vi "Live window-Graph intensity matching.vi"(8 "error in (no error)":errorcluster, 11 "Left/Right":T1) -> (0 "error out":errorcluster)   [LabVIEW 2017]
uses:
  Typedefs/Left-Right enum.ctl
  Globals/gl_Windows Ctrl refs.vi
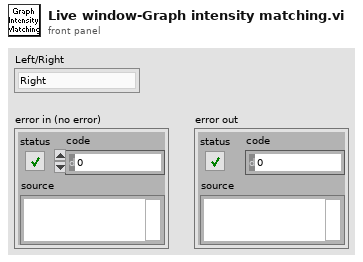
[diagram p1: front panel]
types:
  T1 = typedef "Left-Right enum.ctl" = enum16{"Right", "Left"}
  T2 = typedef "Live window-ctrl refs.ctl" = cluster{"This VI":refnum<vi>, "Pane":refnum<vi>, "Show REF Image Left":refnum<vi>, "Show REF Image Right":refnum<vi>, "Snapshot":refnum<vi>, "Left Image Palette":refnum<vi>, "Right Image Palette":refnum<vi>, "Left Channel":refnum<vi>, "Right Channel":refnum<vi>, "Left image intensity":refnum<vi>, "Right image intensity":refnum<vi>, "Left Image Display":T3, "Right Image Display":T3, "Refresh rate ind (Hz)":refnum<vi>, "Acq rate ind (Hz)":refnum<vi>, "Stop (ind)":refnum<vi>}
  T3 = typedef "Image display ref.ctl" = refnum<vi>
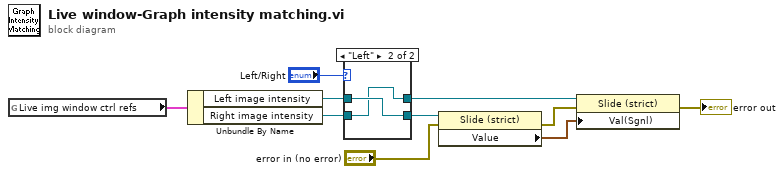
[diagram p0: block diagram]
diagram:
  n1 = global read "gl_Windows Ctrl refs.vi" "Live img window ctrl refs"() -> (w10:T2)
  n2 = Unbundle By Name(w10) -> ("Left image intensity"=w8:refnum<vi>, "Right image intensity"=w6:refnum<vi>)
  n3 = case shown="\"Left\"" "Left/Right" {
    tunnel: w8 -> [w11 w14]
    tunnel: [w12 w14] -> w7
    tunnel: w6 -> [w12 w13]
    tunnel: [w11 w13] -> w5
    frame "Right", Default {
    }
    frame "Left" {
    }
  }
  n4 = property on="Property Node" class="Slide (strict)"(reference=w7, error in="error in (no error)") -> (error out=w3:errorcluster, "Value"=w4:cluster{i16, i16})  [unwired: 1 out]
  n5 = property on="Property Node" class="Slide (strict)"(reference=w5, error in=w3, "Val(Sgnl)"=w4) -> (error out=→"error out":errorcluster)  [unwired: 1 out]
